vi "UI.vi"() -> ()   [LabVIEW 2016, in "DR803M4.lvlib"]
uses:
  DR803M4.lvlib
  Global variable/hold variable.vi
  Global variable/input variable.vi
panel:
  in  "超标留样浓度设置":bool
  out "error out":errorcluster
  in  "VISA资源名称":refnum<visa-resource-name>
  in  "停止":bool
  in  "启动":bool
  in  "门禁":bool
  in  "远程留样":bool
  out "信息簇":T1 {"采样模式选择" items=["定时留样", "时间等比例", "同步留样", "外控留样", "超标留样"]; "启停" items=["停止", "启动"]; "采样器进程" items=["待机"=1, "采样瓶排空"=2, "采样瓶润洗"=5, "进样"=6, "取样"=8, "取样管排空"=9]; "门禁标志" items=["关闭", "打开"]; "远程留样" items=["停止", "留样"]}
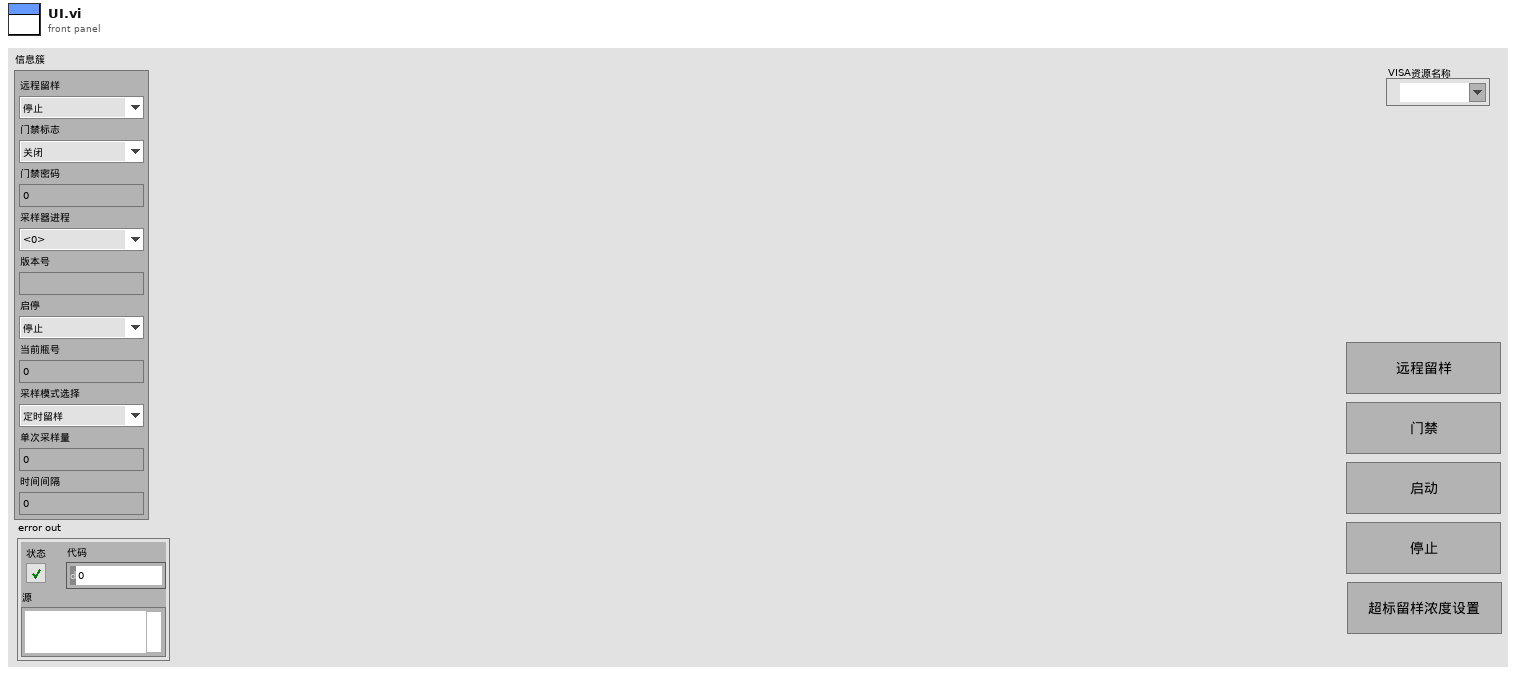
[diagram p1: front panel]
types:
  T1 = cluster{"远程留样":u16, "门禁标志":u16, "门禁密码":u32, "采样器进程":u16, "版本号":string, "启停":u16, "当前瓶号":u16, "采样模式选择":u16, "单次采样量":u16, "时间间隔":u16}
  T2 = cluster{"氨氮超标浓度":dbl, "总磷超标浓度":dbl, "总氮超标浓度":dbl, "CODMn超标浓度":dbl, "CODCr超标浓度":dbl}
  T3 = cluster{"确定":bool, "氨氮超标浓度":dbl, "总磷超标浓度":dbl, "总氮超标浓度":dbl, "CODMn超标浓度":dbl, "CODCr超标浓度":dbl}
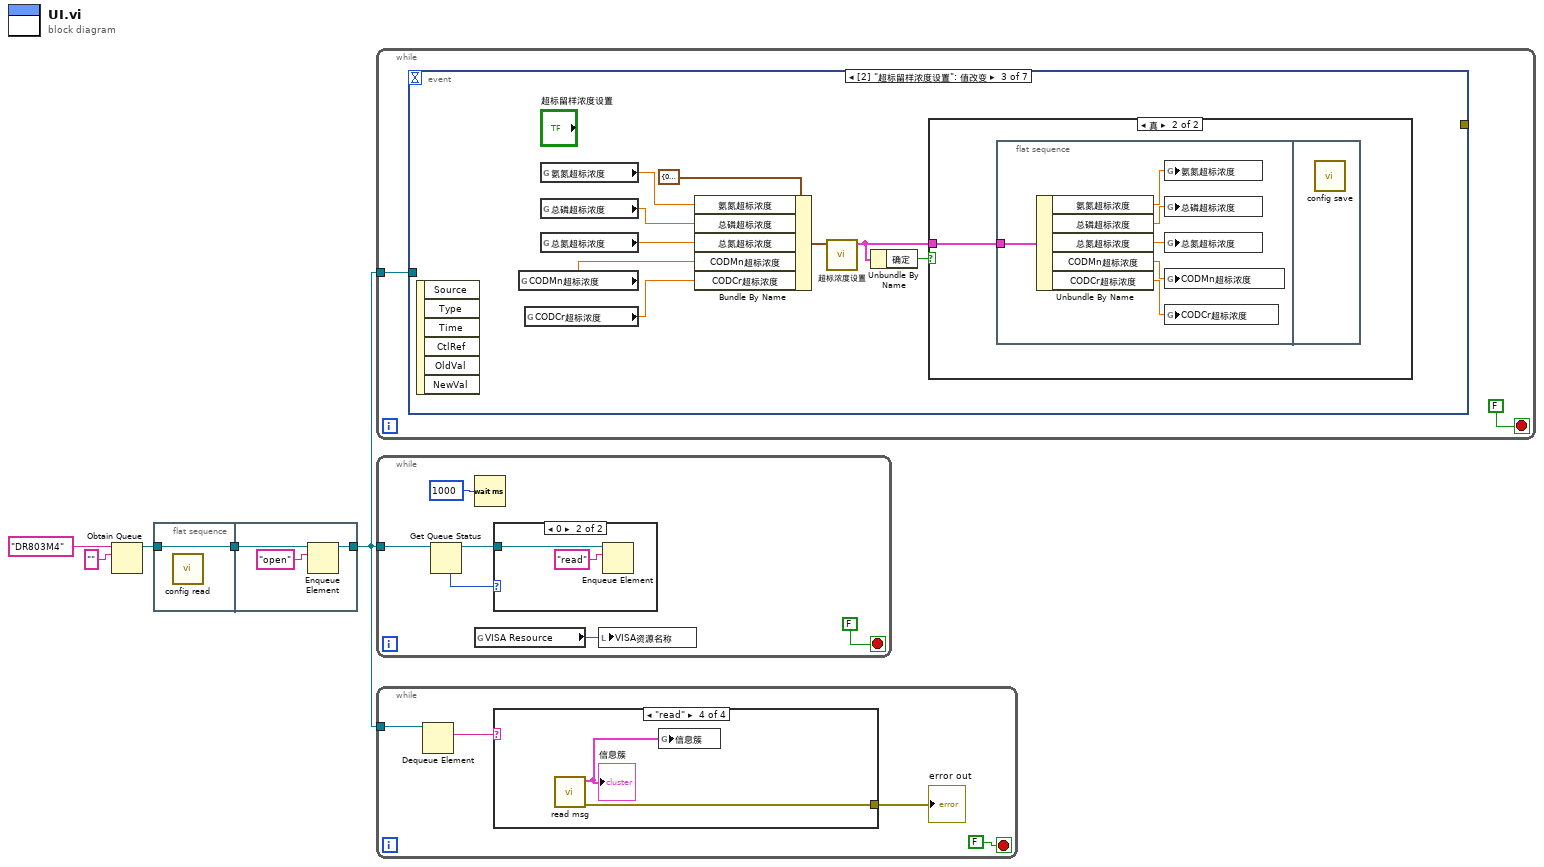
[diagram p0: block diagram]
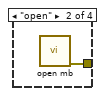
[diagram p4: hidden frame]
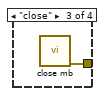
[diagram p5: hidden frame]
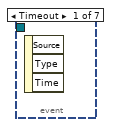
[diagram p6: hidden frame]
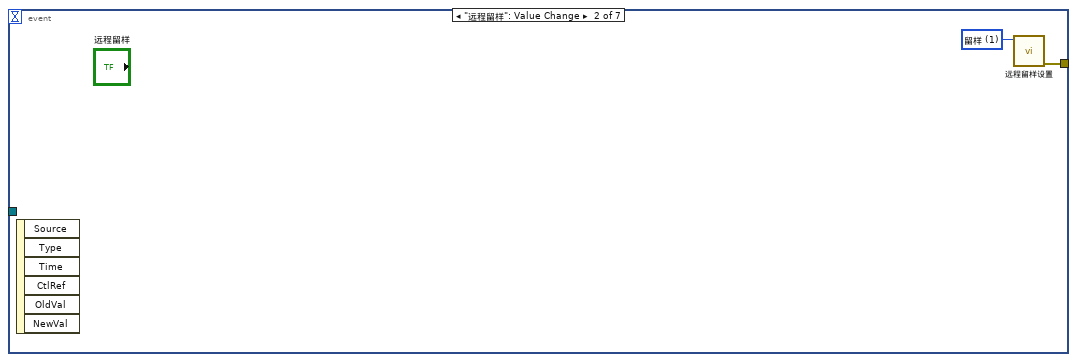
[diagram p7: hidden frame]
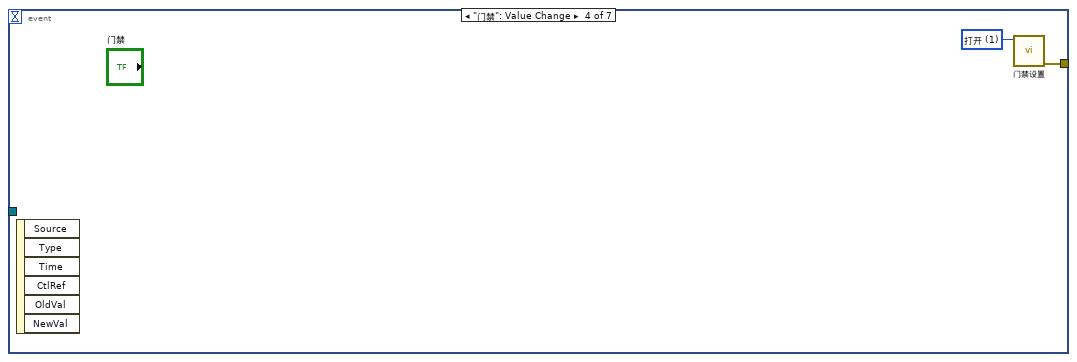
[diagram p9: hidden frame]
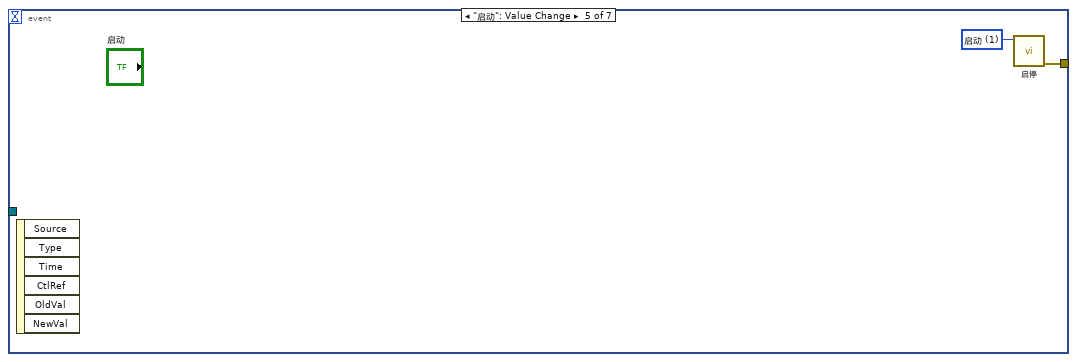
[diagram p10: hidden frame]
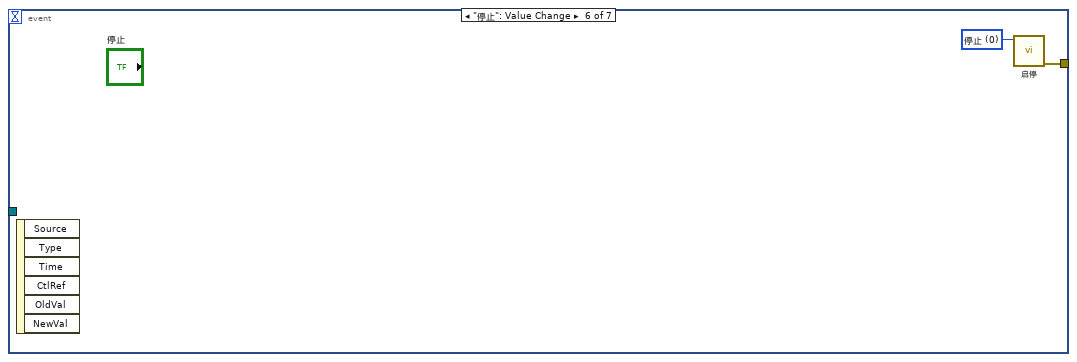
[diagram p11: hidden frame]
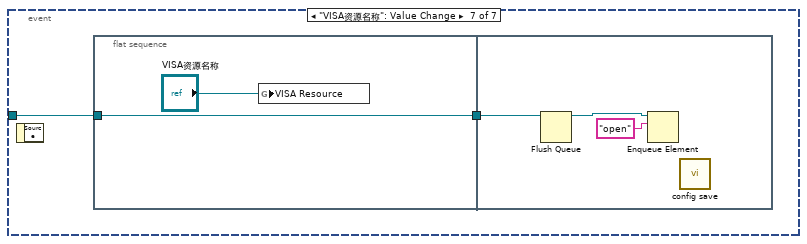
[diagram p12: hidden frame]
diagram:
  n1 = Obtain Queue(name (unnamed)="DR803M4" ("名称（未命名）"), element data type="") -> (queue out=w4:refnum<queue>)  [unwired: 3 in, 2 out]
  n2 = flat-sequence {
    tunnel: w4 -> [w6]
    tunnel: [w6] -> w1
    tunnel: [w8] -> w3
    tunnel: w1 -> [w9]
    frame #0 {
      n3 = call "config read.vi"() -> ()  [unwired: 11 in, 1 out]
    }
    frame #1 {
      n4 = Enqueue Element(queue=w9, element="open" ("元素")) -> (queue out=w8:refnum<queue>)  [unwired: 2 in, 2 out]
    }
  }
  n5 = while {
    tunnel: w3 -> [w10]
    stop <- FALSE stop-if-true
    n6 = event shown="[2] \"超标留样浓度设置\": 值改变" {
      selector: _ -> [_ _ _ _ _ _ _]
      dyn-events: _ -> [_ _ _ _ _ _ _]
      timeout: _ -> [_ _ _ _ _ _ _]
      tunnel: [_ w12 _ w30 w33 w35 _] -> _
      tunnel: w10 -> [_ _ _ _ _ _ w36]
      event Timeout {
        n7 = event-data() -> ()  [unwired: 1 in, 3 out]
      }
      event "远程留样": Value Change {
        w13 = u16 1 items=["停止", "留样"] ("远程留样")
        n8 = event-data() -> ()  [unwired: 1 in, 6 out]
        n9 = call "远程留样设置.vi"("远程留样"=w13) -> ("error out"=w12:errorcluster)  [unwired: 10 in]
      }
      event "超标留样浓度设置": Value Change {
        n10 = event-data() -> ()  [unwired: 1 in, 6 out]
        n11 = global read "hold variable.vi" "CODMn超标浓度"() -> (w17:dbl)
        n12 = global read "hold variable.vi" "CODCr超标浓度"() -> (w16:dbl)
        n13 = global read "hold variable.vi" "氨氮超标浓度"() -> (w20:dbl)
        n14 = global read "hold variable.vi" "总磷超标浓度"() -> (w19:dbl)
        n15 = global read "hold variable.vi" "总氮超标浓度"() -> (w18:dbl)
        n16 = Bundle By Name(cluster=T2 {"氨氮超标浓度"=0.0, "总磷超标浓度"=0.0, "总氮超标浓度"=0.0, "CODMn超标浓度"=0.0, "CODCr超标浓度"=0.0} ("输入"), "氨氮超标浓度"=w20, "总磷超标浓度"=w19, "总氮超标浓度"=w18, "CODMn超标浓度"=w17, "CODCr超标浓度"=w16) -> (w21:T2)
        n17 = call "超标浓度设置.vi"("输入"=w21) -> ("输出"=w14:T3)  [unwired: 10 in]
        n18 = Unbundle By Name(w14) -> ("确定"=w15:bool)
        n19 = case shown="真" w15 {
          tunnel: w14 -> [_ w23]
          frame False {
          }
          frame True {
            n20 = flat-sequence {
              tunnel: w23 -> [w29]
              frame #0 {
                n21 = Unbundle By Name(w29) -> ("氨氮超标浓度"=w28:dbl, "总磷超标浓度"=w27:dbl, "总氮超标浓度"=w26:dbl, "CODMn超标浓度"=w25:dbl, "CODCr超标浓度"=w24:dbl)
                n22 = global write "hold variable.vi" "氨氮超标浓度"(w28) -> ()
                n23 = global write "hold variable.vi" "总磷超标浓度"(w27) -> ()
                n24 = global write "hold variable.vi" "总氮超标浓度"(w26) -> ()
                n25 = global write "hold variable.vi" "CODMn超标浓度"(w25) -> ()
                n26 = global write "hold variable.vi" "CODCr超标浓度"(w24) -> ()
              }
              frame #1 {
                n27 = call "config save.vi"() -> ()  [unwired: 11 in, 1 out]
              }
            }
          }
        }
      }
      event "门禁": Value Change {
        w31 = u16 1 items=["关闭", "打开"] ("门禁标志")
        n28 = event-data() -> ()  [unwired: 1 in, 6 out]
        n29 = call "门禁设置.vi"("门禁标志"=w31) -> ("error out"=w30:errorcluster)  [unwired: 10 in]
      }
      event "启动": Value Change {
        w32 = u16 1 items=["停止", "启动"] ("启停")
        n30 = event-data() -> ()  [unwired: 1 in, 6 out]
        n31 = call "启停.vi"("启停"=w32) -> ("error out"=w33:errorcluster)  [unwired: 10 in]
      }
      event "停止": Value Change {
        w34 = u16 0 items=["停止", "启动"] ("启停")
        n32 = event-data() -> ()  [unwired: 1 in, 6 out]
        n33 = call "启停.vi"("启停"=w34) -> ("error out"=w35:errorcluster)  [unwired: 10 in]
      }
      event "VISA资源名称": Value Change {
        n34 = event-data() -> ()  [unwired: 1 in, 1 out]
        n35 = flat-sequence {
          tunnel: [w38] -> w37
          tunnel: w36 -> [w38]
          tunnel: w37 -> [w41]
          frame #0 {
            n36 = global write "hold variable.vi" "VISA Resource"("VISA资源名称") -> ()
          }
          frame #1 {
            n37 = Flush Queue(queue=w41) -> (queue out=w42:refnum<queue>)  [unwired: 1 in, 2 out]
            n38 = Enqueue Element(queue=w42, element="open" ("元素")) -> ()  [unwired: 2 in, 3 out]
            n39 = call "config save.vi"() -> ()  [unwired: 11 in, 1 out]
          }
        }
      }
    }
  }
  n40 = while {
    tunnel: w3 -> [w45]
    stop <- FALSE stop-if-true
    n41 = Get Queue Status(queue=w45) -> (queue out=w43:refnum<queue>, # elements in queue=w44:i32)  [unwired: 2 in, 6 out]
    n42 = Wait (ms)(milliseconds to wait=u32 1000 ("等待时间（毫秒）")) -> ()  [unwired: 1 out]
    n43 = global read "hold variable.vi" "VISA Resource"() -> (w46:refnum<visa-resource-name>)
    n44 = case shown="0" w44 {
      tunnel: w43 -> [_ w50]
      frame Default {
      }
      frame 0 {
        n45 = Enqueue Element(queue=w50, element="read" ("元素")) -> ()  [unwired: 2 in, 3 out]
      }
    }
    n46 = local write "VISA资源名称"(w46) -> ()
  }
  n47 = while {
    tunnel: w3 -> [w54]
    stop <- FALSE stop-if-true
    n48 = Dequeue Element(queue=w54) -> (element=w53:string)  [unwired: 2 in, 3 out]
    n49 = case shown="\"read\"" w53 {
      tunnel: [_ w55 w56 w58] -> w52
      frame Default {
      }
      frame "open" {
        n50 = call "open mb.vi"() -> ("Error out"=w55:errorcluster)  [unwired: 11 in]
      }
      frame "close" {
        n51 = call "close mb.vi"() -> ("error out"=w56:errorcluster)  [unwired: 11 in]
      }
      frame "read" {
        n52 = call "read msg.vi"() -> ("error out"=w58:errorcluster, "信息簇"=w57:T1)  [unwired: 10 in]
        "信息簇" <- w57
        n53 = global write "input variable.vi" "信息簇"(w57) -> ()
      }
    }
    "error out" <- w52
  }
